vi "Configure Dialog.vi"(8 "Error In":errorcluster, 11 "Open Actor Core FP Msg in":refnum<class "Open Actor Core FP Msg.lvclass">) -> (0 "Error Out":errorcluster, 2 "OK?":bool, 3 "Open Actor Core FP Msg out":refnum<class "Open Actor Core FP Msg.lvclass">)   [LabVIEW 2014, in "CS++BaseActor.lvlib" / "Open Actor Core FP Msg.lvclass"]
doc: "This overrides of this dynamic dispatch VI open the frontpanel to set derived message attributes."
uses:
  Open Actor Core FP Msg.lvclass
  Open Actor Core FP Msg.lvclass/Open Actor Core FP Msg.ctl
panel:
  in  "Cancel":bool
  in  "OK":bool
  in  "Open FP (F)":bool
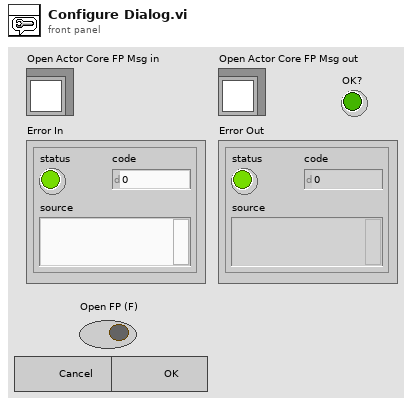
[diagram p1: front panel]
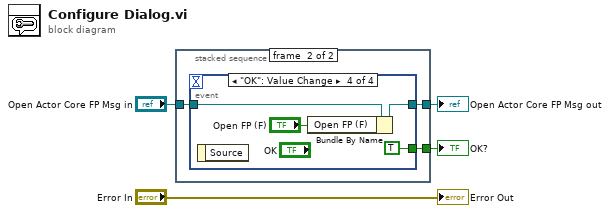
[diagram p0: block diagram]
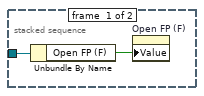
[diagram p2: hidden frame]
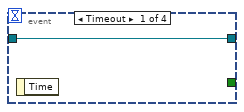
[diagram p3: hidden frame]
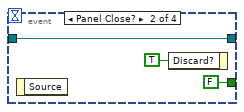
[diagram p4: hidden frame]
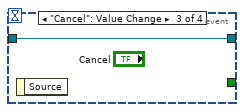
[diagram p5: hidden frame]
diagram:
  n1 = stacked-sequence {
    tunnel: [_ w9] -> w4
    tunnel: "Open Actor Core FP Msg in" -> [w6 w8]
    tunnel: [_ w7] -> w2
    frame #0 {
      n2 = Unbundle By Name(w6) -> ("Open FP (F)"=w5:bool)
      n3 = property on="Open FP (F)" class="Bool (strict)"("Value"=w5) -> ()  [unwired: 2 in, 2 out]
    }
    frame #1 {
      n4 = event shown="[3] \"OK\": Value Change" {
        selector: _ -> [_ _ _ _]
        dyn-events: _ -> [_ _ _ _]
        timeout: _ -> [_ _ _ _]
        tunnel: [w10 w11 w14 w17] -> w9
        tunnel: w8 -> [w10 w11 w14 w18]
        tunnel: [_ FALSE _ TRUE] -> w7
        event Timeout {
          n5 = event-data() -> ()  [unwired: 1 in, 1 out]
        }
        event Panel Close? {
          n6 = event-data() -> ()  [unwired: 1 in, 1 out]
          n7 = event-data("Discard?"=TRUE) -> ()  [unwired: 1 in, 1 out]
        }
        event "Cancel": Value Change {
          n8 = event-data() -> ()  [unwired: 1 in, 1 out]
        }
        event "OK": Value Change {
          n9 = event-data() -> ()  [unwired: 1 in, 1 out]
          n10 = Bundle By Name(cluster=w18, "Open FP (F)"="Open FP (F)") -> (w17:refnum<class "Open Actor Core FP Msg.lvclass">)
        }
      }
    }
  }
  "Open Actor Core FP Msg out" <- w4
  "OK?" <- w2
  "Error Out" <- "Error In"
